vi "svx_Orbit TreeInitialize.vi"(8 "State in":T1={"X Scale"={"Name"="Horizontal", "FString"="%#.2g", "Major Color"=16777238, "Minor Color"=16777216, "Scale Visible"=TRUE, " Label Visible"=TRUE, "Grid Style"=1}, "Y Scale"={"Name"="Vertical", "FString"="%#.2g", "Major Color"=16777238, "Minor Color"=16777216, "Scale Visible"=TRUE, " Label Visible"=TRUE, "Grid Style"=1}, "Plot"={"Point Style"=0, "Line Width"=0, "Line Style"=0, "Plot Color"=9727, "Point/fill"=0}, "Arrow/Crosshair Color"=9727, "Tacho Point Color"=16711680, "Container Bounds"={"Width"=563, "Height"=294}, "Axis Maximum"=10.0, "Probe Angles"={"Angle X"=0.0, "Angle Y"=1.5707963267948966}, "Background Color"=16777226, "Cursor"={"Cursor Point Style"=13, "Cursor Style"=4, "Cursor Line Width"=1, "Cursor Line Style"=0, "Cursor Color"=9727, "Cursor Name Visible"=TRUE, "Cursor Visible"=TRUE, "Cursor Position"={"X"=0.0, "Y"=0.0}, "Cursor Index"=0, "Cursor Lock"=FALSE}, "Elliptical Info"=[], "Legend Visible"=TRUE, "Scale Range Change"=refnum, "Strings[]"={"Custom pair name"=FALSE, "Row Strings []"=[], "Column Strings []"=[]}, "Index"=[{"pair index"=0, "order index"=0}], " Parents Tags"=[], "Children Tags"=[], "Open?"=[], "Label"="", "Legend Width"=120, "Pair Strings Changed?"=FALSE, "Size"=[], "Legend Background"=16777226, "Legend Font"=16777222, "Cursor Release"=refnum, "Autoscale"=TRUE, "Precession Direction"=[], "Item Width"=0, "User Pair Strings []"=[], "Users Order Strings []"=[], "Autoscale Once"=TRUE, "Property Write"=refnum} caption="State" {"Index"."order index" min=0; "Index"."pair index" min=0; "Axis Maximum" min=0.0}, 11 "Tree ref in":refnum<vi>) -> (0 "State out":T1={"X Scale"={"Name"="Horizontal", "FString"="%#.2g", "Major Color"=16777238, "Minor Color"=16777216, "Scale Visible"=TRUE, " Label Visible"=TRUE, "Grid Style"=1}, "Y Scale"={"Name"="Vertical", "FString"="%#.2g", "Major Color"=16777238, "Minor Color"=16777216, "Scale Visible"=TRUE, " Label Visible"=TRUE, "Grid Style"=1}, "Plot"={"Point Style"=0, "Line Width"=0, "Line Style"=0, "Plot Color"=9727, "Point/fill"=0}, "Arrow/Crosshair Color"=9727, "Tacho Point Color"=16711680, "Container Bounds"={"Width"=563, "Height"=294}, "Axis Maximum"=10.0, "Probe Angles"={"Angle X"=0.0, "Angle Y"=1.5707963267948966}, "Background Color"=16777226, "Cursor"={"Cursor Point Style"=13, "Cursor Style"=4, "Cursor Line Width"=1, "Cursor Line Style"=0, "Cursor Color"=9727, "Cursor Name Visible"=TRUE, "Cursor Visible"=TRUE, "Cursor Position"={"X"=0.0, "Y"=0.0}, "Cursor Index"=0, "Cursor Lock"=FALSE}, "Elliptical Info"=[], "Legend Visible"=TRUE, "Scale Range Change"=refnum, "Strings[]"={"Custom pair name"=FALSE, "Row Strings []"=[], "Column Strings []"=[]}, "Index"=[{"pair index"=0, "order index"=0}], " Parents Tags"=[], "Children Tags"=[], "Open?"=[], "Label"="", "Legend Width"=120, "Pair Strings Changed?"=FALSE, "Size"=[], "Legend Background"=16777226, "Legend Font"=16777222, "Cursor Release"=refnum, "Autoscale"=TRUE, "Precession Direction"=[], "Item Width"=0, "User Pair Strings []"=[], "Users Order Strings []"=[], "Autoscale Once"=TRUE, "Property Write"=refnum} caption="State" {"Index"."order index" min=0; "Index"."pair index" min=0; "Axis Maximum" min=0.0}, 3 "Tree ref out":refnum<vi>)   [LabVIEW 2017, in "SVX Orbit.xctl"]
uses:
  <vilib>/addons/_XControls/Orbit Plot/SVX Orbit.xctl
  <vilib>/addons/_XControls/Orbit Plot/subVIs/svx_Orbit Internal State.ctl
  <vilib>/addons/_XControls/Orbit Plot/subVIs/svx_Orbit Bounds.ctl
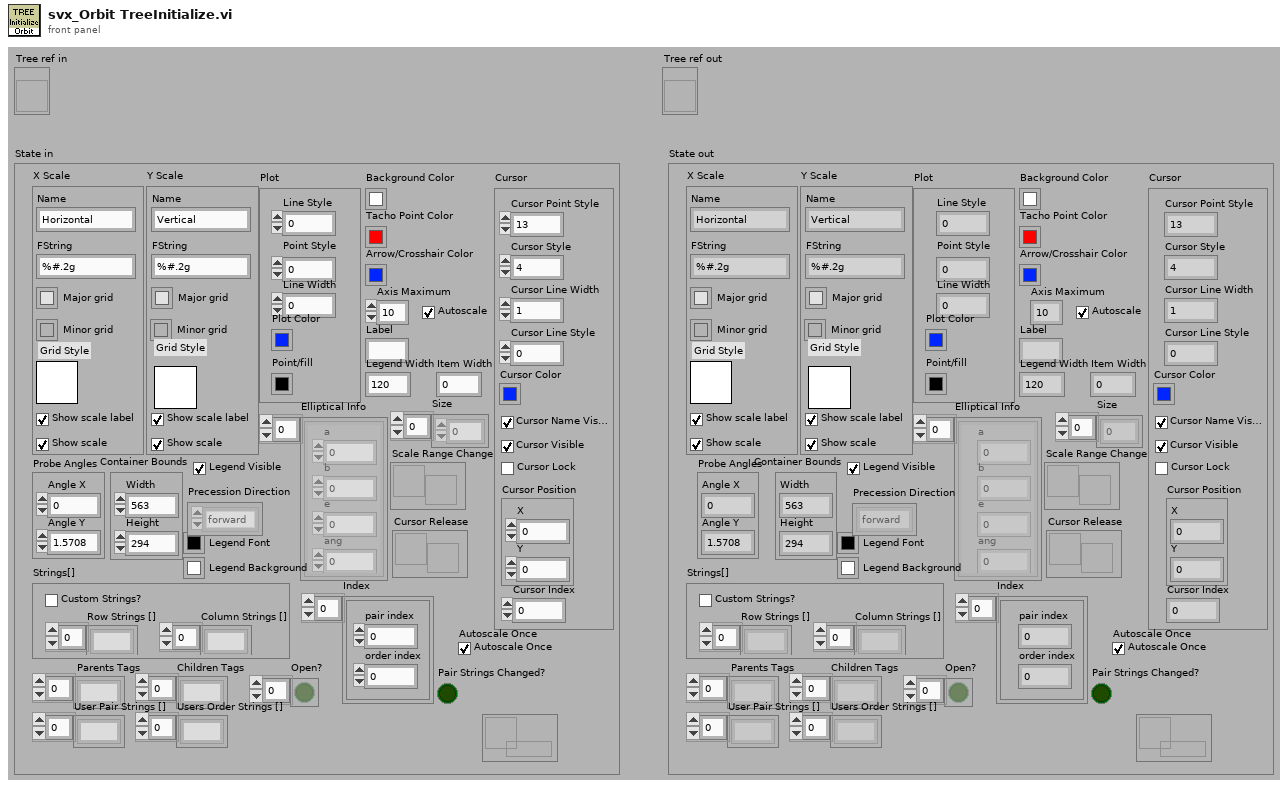
[diagram p1: front panel]
types:
  T1 = typedef "SVX Orbit.xctl/svx_Orbit Internal State.ctl" = cluster{"X Scale":cluster{"Name":string, "FString":string, "Major Color":u32, "Minor Color":u32, "Scale Visible":bool, " Label Visible":bool, "Grid Style":u16}, "Y Scale":cluster{"Name":string, "FString":string, "Major Color":u32, "Minor Color":u32, "Scale Visible":bool, " Label Visible":bool, "Grid Style":u16}, "Plot":cluster{"Point Style":u8, "Line Width":u8, "Line Style":u8, "Plot Color":u32, "Point/fill":u32}, "Arrow/Crosshair Color":u32, "Tacho Point Color":u32, "Container Bounds":T2, "Axis Maximum":dbl, "Probe Angles":cluster{"Angle X":dbl, "Angle Y":dbl}, "Background Color":u32, "Cursor":cluster{"Cursor Point Style":u8, "Cursor Style":u8, "Cursor Line Width":u8, "Cursor Line Style":u8, "Cursor Color":u32, "Cursor Name Visible":bool, "Cursor Visible":bool, "Cursor Position":cluster{"X":dbl, "Y":dbl}, "Cursor Index":i32, "Cursor Lock":bool}, "Elliptical Info":cluster{"a":dbl, "b":dbl, "e":dbl, "ang":dbl}[], "Legend Visible":bool, "Scale Range Change":refnum<user-event>, "Strings[]":cluster{"Custom pair name":bool, "Row Strings []":string[], "Column Strings []":string[]}, "Index":cluster{"pair index":i32, "order index":i32}[], " Parents Tags":string[], "Children Tags":string[], "Open?":bool[], "Label":string, "Legend Width":u32, "Pair Strings Changed?":bool, "Size":i32[], "Legend Background":u32, "Legend Font":u32, "Cursor Release":refnum<user-event>, "Autoscale":bool, "Precession Direction":enum16{"forward", "backward"}[], "Item Width":u32, "User Pair Strings []":string[], "Users Order Strings []":string[], "Autoscale Once":bool, "Property Write":refnum<queue>}
  T2 = typedef "SVX Orbit.xctl/svx_Orbit Bounds.ctl" = cluster{"Width":u32, "Height":u32}
  T3 = enum16{"User-specified Font", "Application Font", "System Font", "Dialog Font"}
  T4 = cluster{"Left Cell String":string, "Child Text":string[], "Child Tag":string, "Item Indent":i32, "Child Only?":bool, "Glyph Index":i32}
  T5 = cluster{"Left Cell String":string, "Child Text":string[], "Child Tag":string, "Item Indent":i32, "Child Only?":bool, "Glyph Index":i32}[]
  T6 = cluster{"left":i16, "top":i16, "right":i16, "bottom":i16}
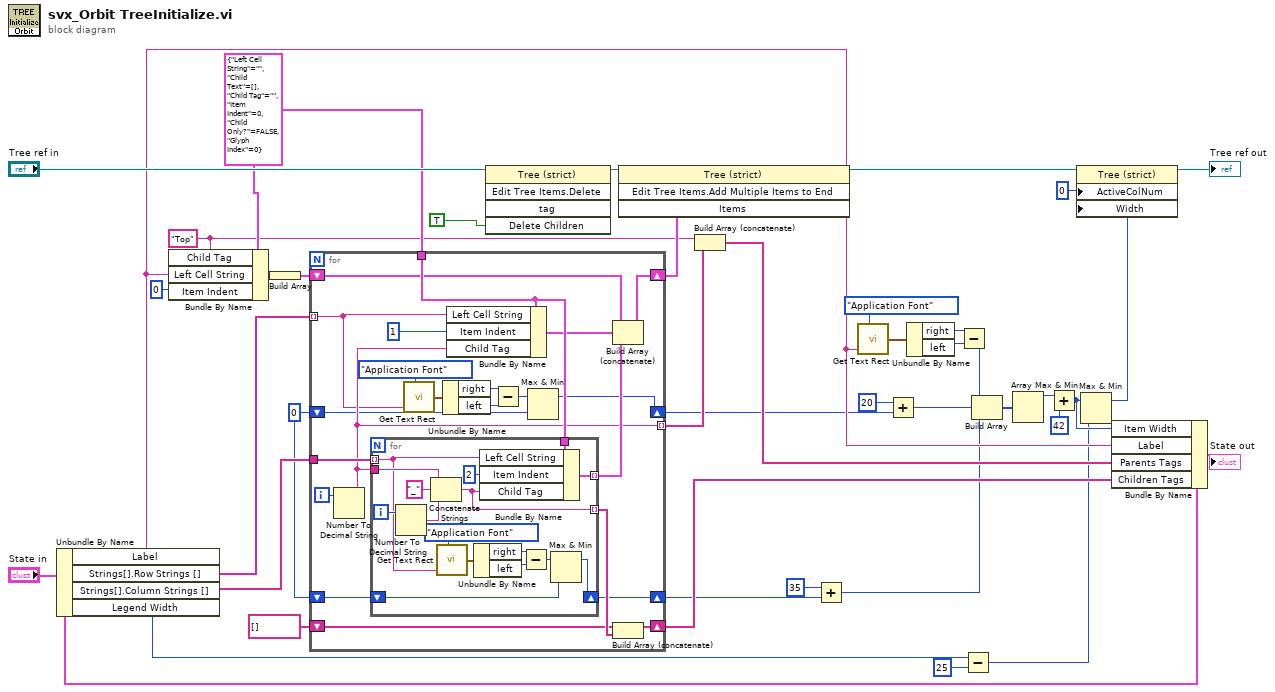
[diagram p0: block diagram]
diagram:
  w19 = u32 0
  w30 = "Top" ("Child Tag")
  w37 = T4 {"Left Cell String"="", "Child Text"=[], "Child Tag"="", "Item Indent"=0, "Child Only?"=FALSE, "Glyph Index"=0} ("element")
  n1 = Unbundle By Name("State in") -> ("Label"=w20:string, "Strings[].Row Strings []"=w26:string[], "Strings[].Column Strings []"=w25:string[], "Legend Width"=w2:u32)
  n2 = Bundle By Name(cluster=w37, "Child Tag"=w30, "Left Cell String"=w20, "Item Indent"=0) -> (w36:T4)
  n3 = Build Array(w36) -> (w35:T5)
  n4 = for {
    tunnel: w37 -> [w62]
    tunnel: w26 -> [w48] mode=indexing
    shift-right: [w58] -> w32
    shift-left: w35 -> [w59]
    tunnel: w25 -> [w63]
    shift-right: [w53] -> w28
    shift-left: string[] [] -> [w54]
    tunnel: [w52] -> w29 mode=indexing
    shift-right: [w44] -> w17
    shift-left: w19 -> [w45]
    shift-right: [w43] -> w15
    shift-left: w19 -> [w42]
    i -> [w56]
    n5 = Number To Decimal String(number=w56) -> (decimal integer string=w52:string)  [unwired: 1 in]
    n6 = for {
      tunnel: w63 -> [w66] mode=indexing
      tunnel: w62 -> [w79]
      tunnel: [w77] -> w57 mode=indexing
      tunnel: [w75] -> w55 mode=indexing
      tunnel: w52 -> [w74]
      shift-right: [w64] -> w43
      shift-left: w42 -> [w65]
      i -> [w73]
      n7 = Number To Decimal String(number=w73) -> (decimal integer string=w72:string)  [unwired: 1 in]
      n8 = Concatenate Strings(w74, "_" ("string"), w72) -> (w75:string)
      n9 = call <vilib>:"Get Text Rect.vi"("desired font(Application)"=T3."Application Font", "text"=w66) -> ("rect"=w69:T6)  [unwired: 7 in]
      n10 = Unbundle By Name(w69) -> ("right"=w70:i16, "left"=w71:i16)
      n11 = Bundle By Name(cluster=w79, "Left Cell String"=w66, "Item Indent"=2, "Child Tag"=w75) -> (w77:T4)
      n12 = Subtract(x=w70, y=w71) -> (x-y=w67:i16)
      n13 = Max & Min(x=w67, y=w65) -> (max(x,y)=w64:u32)  [unwired: 1 out]
    }
    n14 = call <vilib>:"Get Text Rect.vi"("desired font(Application)"=T3."Application Font", "text"=w48) -> ("rect"=w50:T6)  [unwired: 7 in]
    n15 = Unbundle By Name(w50) -> ("right"=w51:i16, "left"=w47:i16)
    n16 = Bundle By Name(cluster=w62, "Left Cell String"=w48, "Item Indent"=1, "Child Tag"=w52) -> (w60:T4)
    n17 = Subtract(x=w51, y=w47) -> (x-y=w49:i16)
    n18 = Max & Min(x=w49, y=w45) -> (max(x,y)=w44:u32)  [unwired: 1 out]
    n19 = Build Array (concatenate)(w59, w60, w57) -> (w58:T5)
    n20 = Build Array (concatenate)(w54, w55) -> (w53:string[])
  }
  n21 = invoke on="Invoke Node" class="Tree (strict)" method="Edit Tree Items.Delete"(reference="Tree ref in", "Delete Children"=TRUE ("Delete Children?")) -> (reference out=w33:refnum<vi>)  [unwired: 3 in, 4 out]
  n22 = invoke on="Invoke Node" class="Tree (strict)" method="Edit Tree Items.Add Multiple Items to End"(reference=w33, "Items"=w32) -> (reference out=w7:refnum<vi>)  [unwired: 2 in, 3 out]
  n23 = Build Array (concatenate)(w30, w29) -> (w27:string[])
  n24 = Add(x=u32 35, y=w15) -> (x+y=w12:u32)
  n25 = call <vilib>:"Get Text Rect.vi"("desired font(Application)"=T3."Application Font", "text"=w20) -> ("rect"=w24:T6)  [unwired: 7 in]
  n26 = Add(x=u32 20, y=w17) -> (x+y=w14:u32)
  n27 = Unbundle By Name(w24) -> ("right"=w23:i16, "left"=w22:i16)
  n28 = Subtract(x=w23, y=w22) -> (x-y=w13:i16)
  n29 = Subtract(x=w2, y=u32 25) -> (x-y=w1:u32)
  n30 = Build Array(w13, w14, w12) -> (w9:u32[])
  n31 = Array Max & Min(array=w9) -> (max value=w10:u32)  [unwired: 3 out]
  n32 = Add(x=w10, y=u32 42) -> (x+y=w4:u32)
  n33 = Max & Min(x=w4, y=w1) -> (max(x,y)=w6:u32)  [unwired: 1 out]
  n34 = property class="Tree (strict)"(reference=w7, "ActiveColNum"=0 ("Active Cell:Active Column Number"), "Width"=w6) -> (reference out=→"Tree ref out":refnum<vi>)  [unwired: 1 in, 1 out]
  n35 = Bundle By Name(cluster="State in", "Item Width"=w4, "Label"=w20, "Parents Tags"=w27, "Children Tags"=w28) -> (→"State out":T1)
